vi "PPMS2 Current to Field (Oe).vi"(8 "error in (no error)":errorcluster, 10 "Current (A)":dbl, 11 "instrument.PPMS2 in":refnum<class "instrument.PPMS2.lvclass">) -> (0 "error out":errorcluster, 2 "Field (Oe)":dbl, 3 "instrument.PPMS2 out":refnum<class "instrument.PPMS2.lvclass">)   [LabVIEW 2016, in "instrument.PPMS2.lvclass"]
uses:
  instrument.PPMS2.lvclass
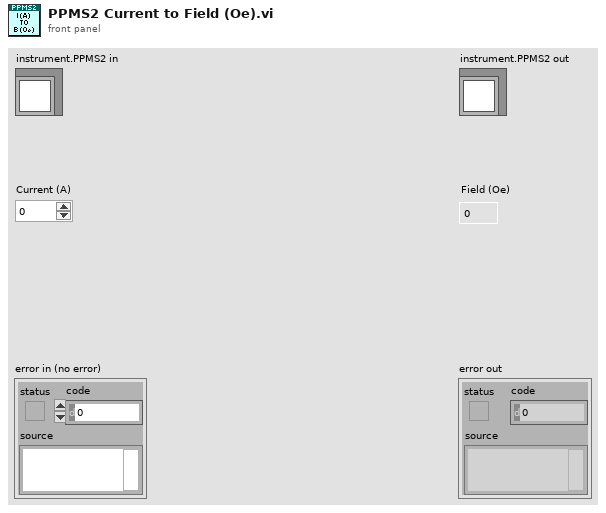
[diagram p1: front panel]
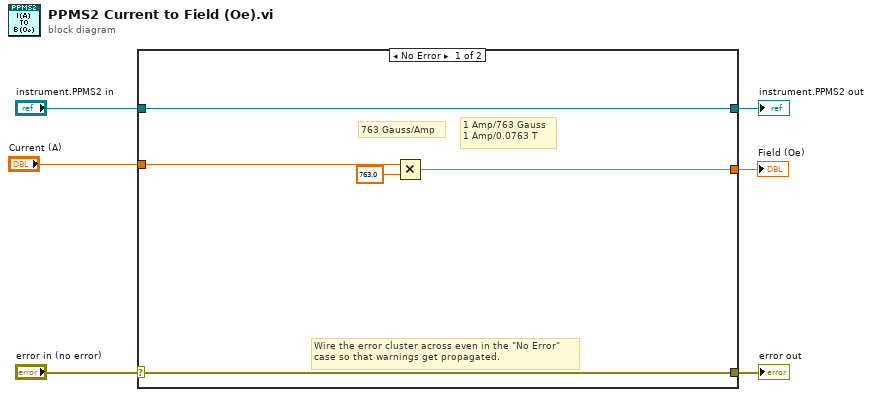
[diagram p0: block diagram]
diagram:
  n1 = case shown="No Error" "error in (no error)" {
    selector: "error in (no error)" -> [w10 w13]
    tunnel: [w10 w13] -> w5
    tunnel: [w11 w12] -> w3
    tunnel: "instrument.PPMS2 in" -> [w11 w12]
    tunnel: "Current (A)" -> [w9 _]
    tunnel: [w7 _] -> w1
    frame No Error {
      # "1 Amp/763 Gauss\n1 Amp/0.0763 T"
      # "763 Gauss/Amp"
      # "Wire the error cluster across even in the \"No Error\"\ncase so that warnings get propagated."
      n2 = Multiply(x=w9, y=763.0) -> (x*y=w7:dbl)
    }
    frame Error {
    }
  }
  "error out" <- w5
  "instrument.PPMS2 out" <- w3
  "Field (Oe)" <- w1
